vi "getAxisBounds.vi"(10 "Active X Scale":i32, 11 "XYGraph in":refnum<vi>) -> (0 "YMapping":enum8{"Lin", "Log"}(ring)=enum."Log", 1 "Ybounds":T1, 2 "XMapping":enum8{"Lin", "Log"}(ring)=enum."Log", 3 "Xbounds":T1)   [LabVIEW 2013]
uses:
  minAndMax.ctl
  AutoManualNumber.ctl
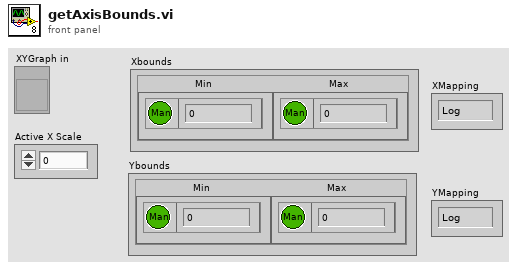
[diagram p1: front panel]
types:
  T1 = typedef "minAndMax.ctl" = cluster{"Min":T2, "Max":T2}
  T2 = typedef "AutoManualNumber.ctl" = cluster{"Auto":bool, "Value":dbl}
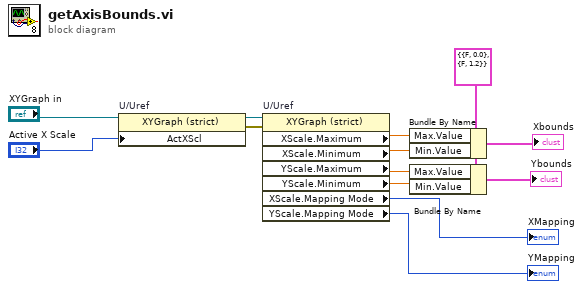
[diagram p0: block diagram]
diagram:
  w11 = T1 {"Min"={"Auto"=FALSE, "Value"=0.0}, "Max"={"Auto"=FALSE, "Value"=1.2}} ("U/UrefBounds")
  n1 = property on="U/Uref" class="XYGraph (strict)"(reference="XYGraph in", "ActXScl"="Active X Scale") -> (reference out=w9:refnum<vi>, error out=w7:errorcluster)  [unwired: 1 in]
  n2 = property on="U/Uref" class="XYGraph (strict)"(reference=w9, error in=w7) -> ("XScale.Maximum"=w5:dbl, "XScale.Minimum"=w6:dbl, "YScale.Maximum"=w12:dbl, "YScale.Minimum"=w1:dbl, "XScale.Mapping Mode"=→"XMapping":u8, "YScale.Mapping Mode"=→"YMapping":u8)  [unwired: 2 out]
  n3 = Bundle By Name(cluster=w11, "Max.Value"=w5, "Min.Value"=w6) -> (→"Xbounds":T1)
  n4 = Bundle By Name(cluster=w11, "Max.Value"=w12, "Min.Value"=w1) -> (→"Ybounds":T1)
